vi "User Config_Main.vi"(8 "Login Status":string, 9 "User Type":string, 11 "Path":path=path "E:/labview code/project user login/test1.txt") -> ()   [LabVIEW 2023]
panel:
  in  "Modify":bool
  in  "Exit":bool
  in  "delete":bool
  in  "Add Button":bool
  # "In-Hous Part Data Retrieval System"
  # "User Setting Screen"
  # "SOFTWARE DEVELOPED BY:-COSMO INSTRUMENTS INDIA PVT. LTD."
  # "SOFTWAERE DEVELOPED BY:-SMO INSTRUMENTS INDIA PVT. LTD."
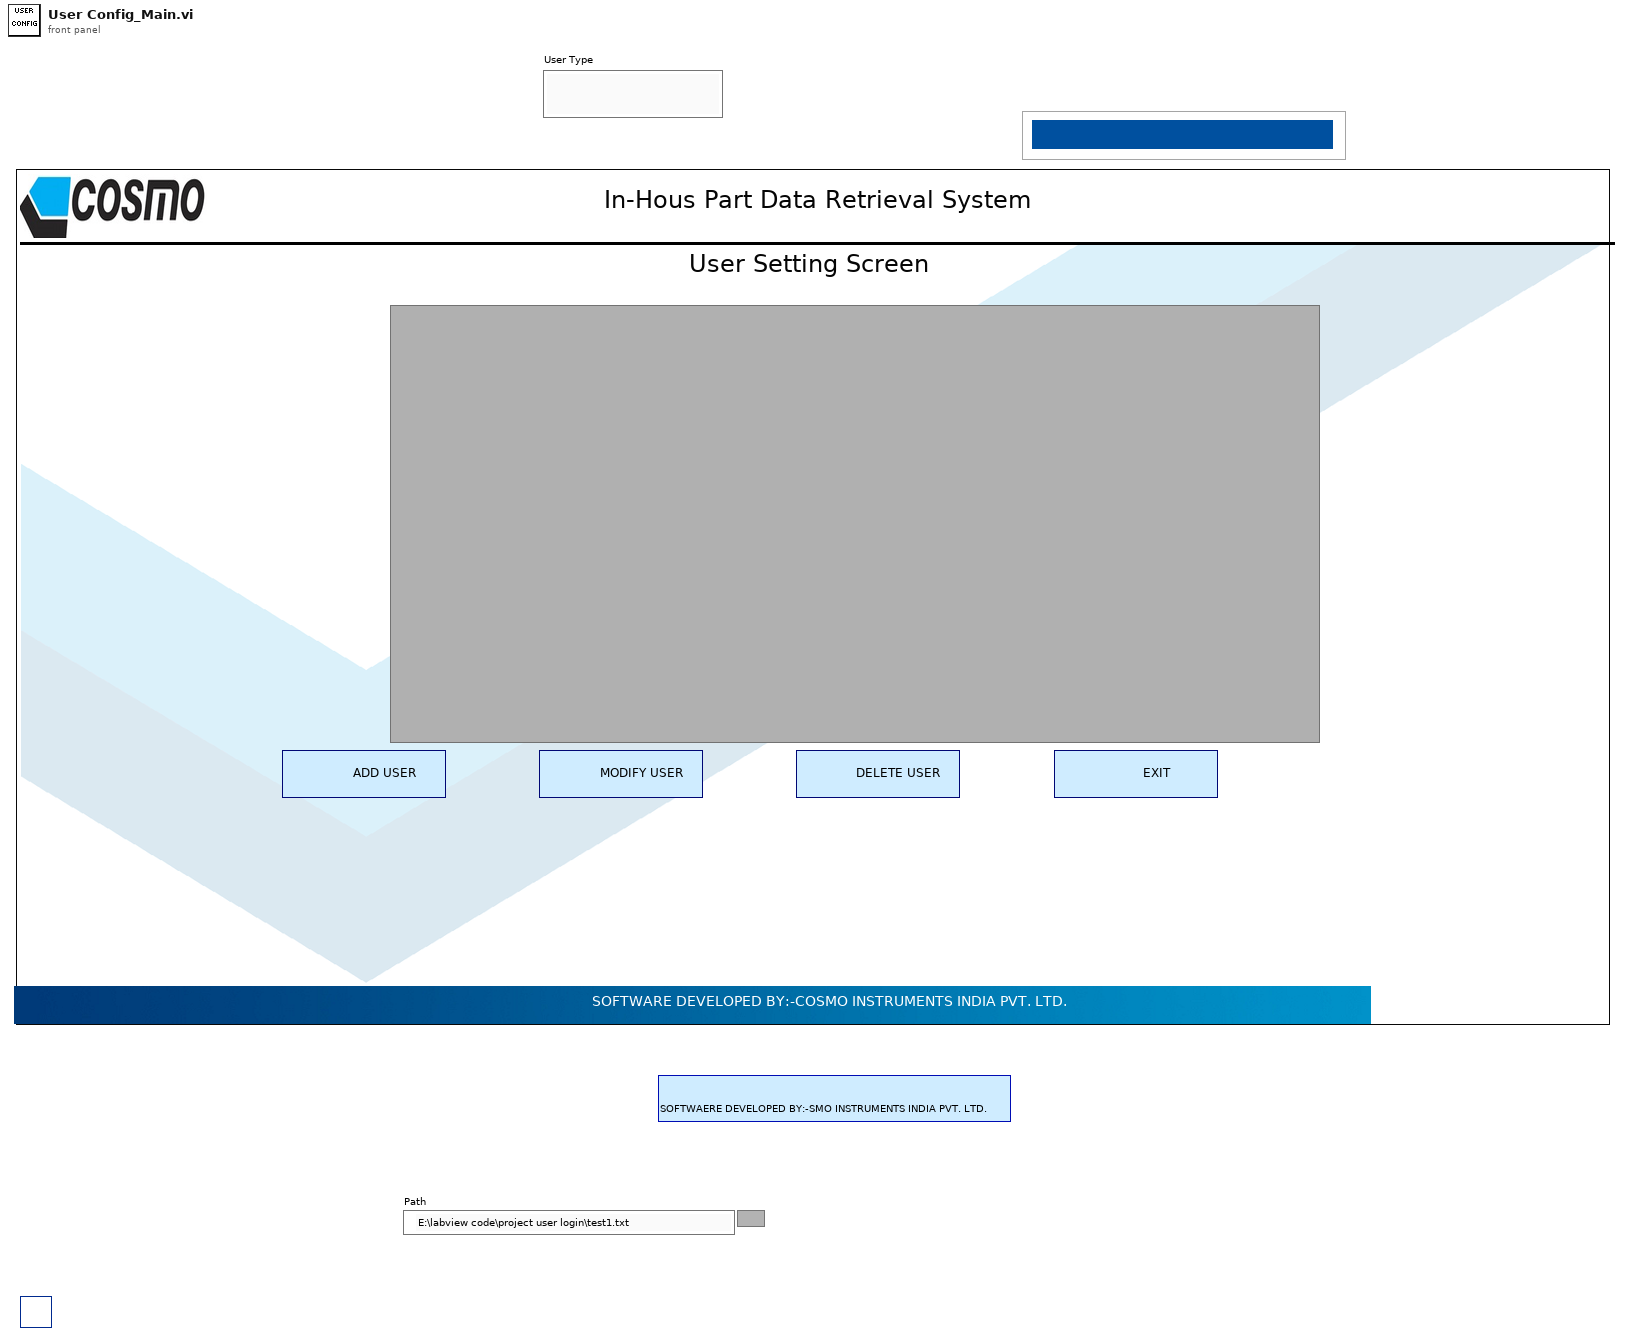
[diagram p1: front panel]
types:
  T1 = enum32{"Bad", "Idle", "Run top level", "Running"}
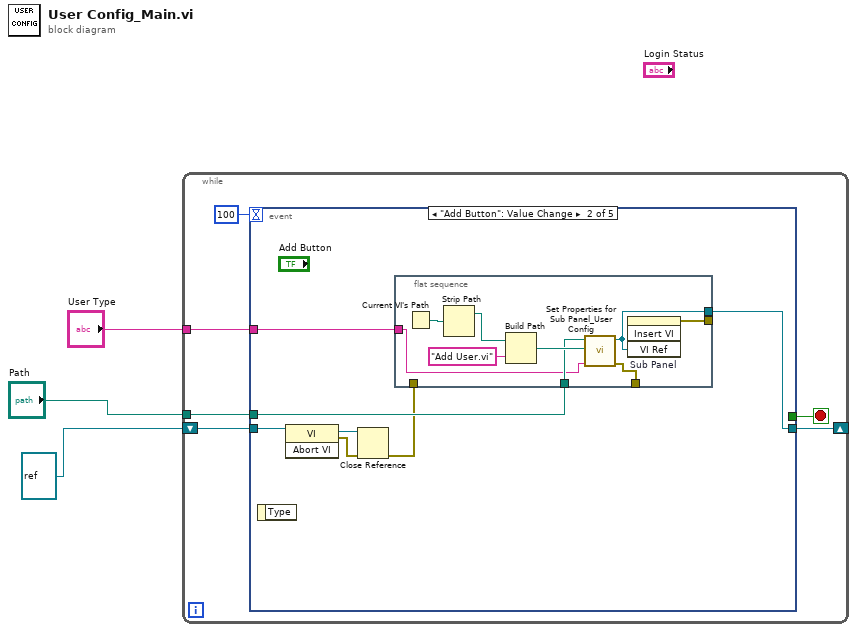
[diagram p0: block diagram]
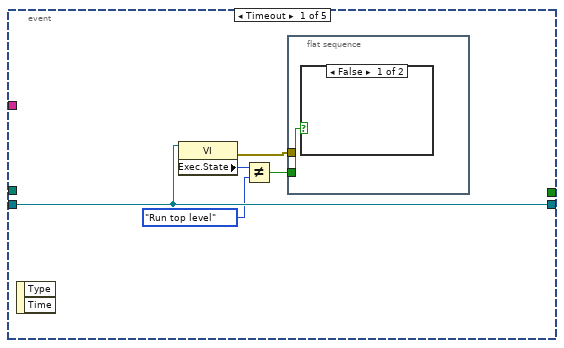
[diagram p2: hidden frame]
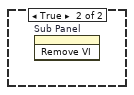
[diagram p3: hidden frame]
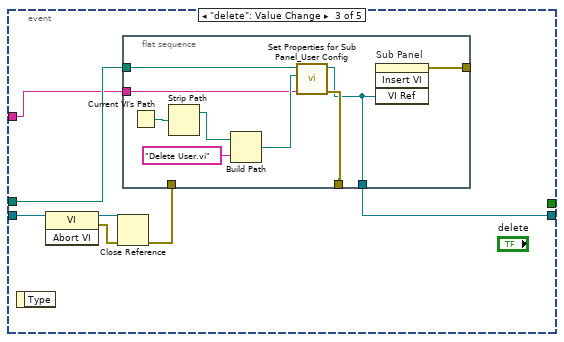
[diagram p4: hidden frame]
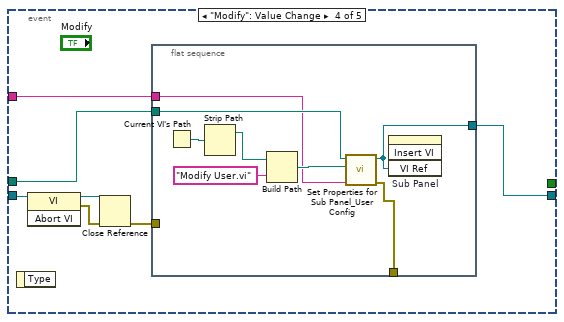
[diagram p5: hidden frame]
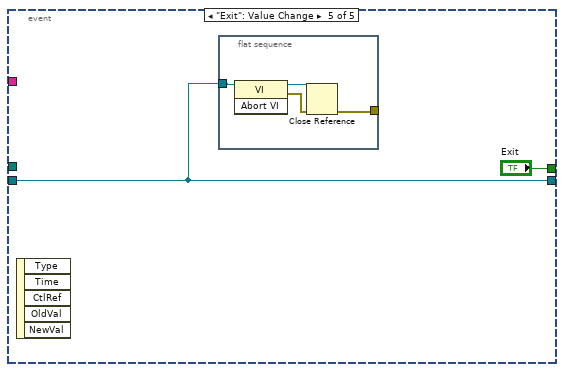
[diagram p6: hidden frame]
diagram:
  n1 = while {
    tunnel: "Path" -> [w8]
    shift-right: [w7] -> _
    shift-left: refnum<vi> refnum ("vi reference") -> [w6]
    tunnel: "User Type" -> [w4]
    stop <- w9 stop-if-true
    n2 = event shown="[1] \"Add Button\": Value Change" {
      selector: _ -> [_ _ _ _ _]
      dyn-events: _ -> [_ _ _ _ _]
      timeout: 100 -> [_ _ _ _ _]
      tunnel: [_ _ _ _ "Exit"] -> w9
      tunnel: w8 -> [_ w22 w38 w53 _]
      tunnel: [w14 w20 w36 w54 w63] -> w7
      tunnel: w6 -> [w14 w18 w35 w51 w63]
      tunnel: w4 -> [_ w21 w37 w52 _]
      event Timeout {
        n3 = event-data() -> ()  [unwired: 1 in, 2 out]
        n4 = property class="VI"(reference=w14) -> (error out=w10:errorcluster, "Exec.State"=w13:T1)  [unwired: 1 in, 1 out]
        n5 = Not Equal?(x=w13, y=T1."Run top level" ("Execution:State")) -> (x != y?=w11:bool)
        n6 = flat-sequence {
          tunnel: w11 -> [w15]
          tunnel: w10 -> [_]
          frame #0 {
            n7 = case shown="False" w15 {
              frame False {
              }
              frame True {
                n8 = invoke on="Sub Panel" class="SubPanel" method="Remove VI"() -> ()  [unwired: 3 in, 3 out]
              }
            }
          }
        }
      }
      event "Add Button": Value Change {
        n9 = event-data() -> ()  [unwired: 1 in, 1 out]
        n10 = invoke class="VI" method="Abort VI"(reference=w18) -> (reference out=w16:refnum<vi>, error out=w19:errorcluster)  [unwired: 2 in, 1 out]
        n11 = Close Reference(reference=w16, error in (no error)=w19) -> (error out=w17:errorcluster)
        n12 = flat-sequence {
          tunnel: w22 -> [w27]
          tunnel: [w26] -> _
          tunnel: [w25] -> _
          tunnel: w21 -> [w24]
          tunnel: [w23] -> w20
          tunnel: w17 -> [_]
          frame #0 {
            n13 = Current VI's Path() -> (path=w31:path)
            n14 = Strip Path(path=w31) -> (stripped path=w30:path)  [unwired: 1 out]
            n15 = Build Path(base path=w30, name or relative path="Add User.vi") -> (appended path=w28:path)
            n16 = call "Set Properties for Sub Panel_User Config.vi"("User Type"=w24, "vi path"=w28, "Path"=w27) -> ("error out"=w25:errorcluster, "VI out"=w23:refnum<vi>)  [unwired: 7 in]
            n17 = invoke on="Sub Panel" class="SubPanel" method="Insert VI"("VI Ref"=w23) -> (error out=w26:errorcluster)  [unwired: 3 in, 3 out]
          }
        }
      }
      event "delete": Value Change {
        n18 = event-data() -> ()  [unwired: 1 in, 1 out]
        n19 = invoke class="VI" method="Abort VI"(reference=w35) -> (reference out=w33:refnum<vi>, error out=w34:errorcluster)  [unwired: 2 in, 1 out]
        n20 = Close Reference(reference=w33, error in (no error)=w34) -> (error out=w32:errorcluster)
        n21 = flat-sequence {
          tunnel: w38 -> [w47]
          tunnel: w37 -> [w42]
          tunnel: [w41] -> _
          tunnel: [w40] -> _
          tunnel: [w39] -> w36
          tunnel: w32 -> [_]
          frame #0 {
            n22 = Current VI's Path() -> (path=w46:path)
            n23 = Strip Path(path=w46) -> (stripped path=w45:path)  [unwired: 1 out]
            n24 = Build Path(base path=w45, name or relative path="Delete User.vi") -> (appended path=w43:path)
            n25 = call "Set Properties for Sub Panel_User Config.vi"("User Type"=w42, "vi path"=w43, "Path"=w47) -> ("error out"=w40:errorcluster, "VI out"=w39:refnum<vi>)  [unwired: 7 in]
            n26 = invoke on="Sub Panel" class="SubPanel" method="Insert VI"("VI Ref"=w39) -> (error out=w41:errorcluster)  [unwired: 3 in, 3 out]
          }
        }
      }
      event "Modify": Value Change {
        n27 = event-data() -> ()  [unwired: 1 in, 1 out]
        n28 = invoke class="VI" method="Abort VI"(reference=w51) -> (reference out=w50:refnum<vi>, error out=w49:errorcluster)  [unwired: 2 in, 1 out]
        n29 = Close Reference(reference=w50, error in (no error)=w49) -> (error out=w48:errorcluster)
        n30 = flat-sequence {
          tunnel: [w62] -> w54
          tunnel: w53 -> [w61]
          tunnel: w52 -> [w56]
          tunnel: [w55] -> _
          tunnel: w48 -> [_]
          frame #0 {
            n31 = Current VI's Path() -> (path=w60:path)
            n32 = Strip Path(path=w60) -> (stripped path=w59:path)  [unwired: 1 out]
            n33 = Build Path(base path=w59, name or relative path="Modify User.vi") -> (appended path=w57:path)
            n34 = call "Set Properties for Sub Panel_User Config.vi"("User Type"=w56, "vi path"=w57, "Path"=w61) -> ("error out"=w55:errorcluster, "VI out"=w62:refnum<vi>)  [unwired: 7 in]
            n35 = invoke on="Sub Panel" class="SubPanel" method="Insert VI"("VI Ref"=w62) -> ()  [unwired: 3 in, 4 out]
          }
        }
      }
      event "Exit": Value Change {
        n36 = event-data() -> ()  [unwired: 1 in, 5 out]
        n37 = flat-sequence {
          tunnel: w63 -> [w67]
          tunnel: [w65] -> _
          frame #0 {
            n38 = invoke class="VI" method="Abort VI"(reference=w67) -> (reference out=w68:refnum<vi>, error out=w66:errorcluster)  [unwired: 2 in, 1 out]
            n39 = Close Reference(reference=w68, error in (no error)=w66) -> (error out=w65:errorcluster)
          }
        }
      }
    }
  }
